vi "DidInit.vi"(8 "ErrorArray":errorcluster[](array[cluster]), 10 "Init?":bool, 11 "Bus":refnum<class "Bus.lvclass">) -> (0 "ErrorArray":errorcluster[](array[cluster]), 3 "Bus":refnum<class "Bus.lvclass">)   [LabVIEW 2014, in "Bus_class.lvlib"]
uses:
  Bus_class.lvlib
  Bus.lvclass
  Typedefs/clDidInit.ctl
  Typedefs/clUserEventType.ctl
  <userlib>/NIST/NISTErrorLib/NISTErrorLib.lvlib
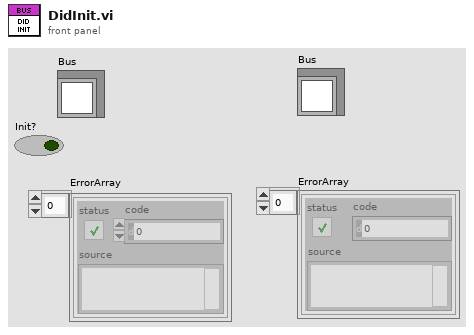
[diagram p1: front panel]
types:
  T1 = typedef "Bus_class.lvlib/clUserEventType.ctl" = cluster{"BusNumber":i8, "Data":variant}
  T2 = typedef "Bus_class.lvlib/clDidInit.ctl" = cluster{"Bus":refnum<vi>, "Init?":bool}
  T3 = typedef "Bus_class.lvlib/clBroadcastEvents.ctl" = cluster{"DidInit":refnum<user-event>, "DidStop":refnum<user-event>}
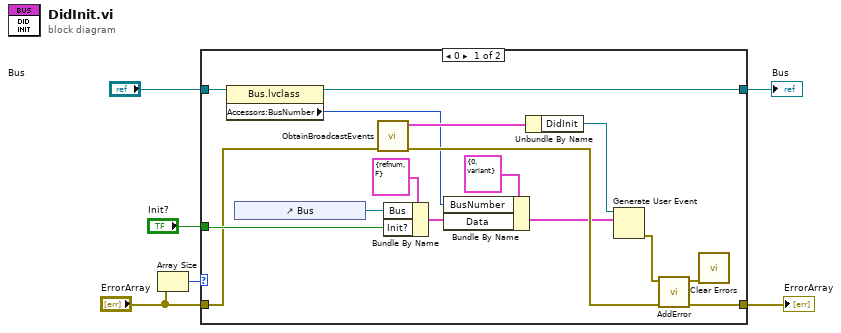
[diagram p0: block diagram]
diagram:
  n1 = Array Size(array="ErrorArray") -> (size(s)=w5:i32)
  n2 = case shown="0" w5 {
    tunnel: "Init?" -> [w19 _]
    tunnel: "ErrorArray" -> [w18 w24]
    tunnel: [w14 w24] -> w3
    tunnel: "Bus" -> [w13 w23]
    tunnel: [w9 w23] -> w1
    frame 0 {
      n3 = property class="Bus.lvclass"(reference=w13) -> (reference out=w9:refnum<class "Bus.lvclass">, "Accessors:BusNumber"=w8:u8)  [unwired: 1 in, 1 out]
      n4 = control-ref of="Bus"() -> (w12:refnum<vi>)
      n5 = call "ObtainBroadcastEvents.vi"("ErrorArray"=w18) -> ("ErrorArray"=w17:errorcluster[], "BusBroadcast"=w22:T3)  [unwired: 9 in]
      n6 = Bundle By Name(cluster=T2 {"Bus"=refnum, "Init?"=FALSE} ("clBusDidInit"), "Bus"=w12, "Init?"=w19) -> (w10:T2)
      n7 = Bundle By Name(cluster=T1 {"BusNumber"=0, "Data"=variant} ("clEventType"), "BusNumber"=w8, "Data"=w10) -> (w7:T1)
      n8 = Unbundle By Name(w22) -> ("DidInit"=w21:refnum<user-event>)
      n9 = Generate User Event(user event=w21, event data cluster=w7) -> (error out=w16:errorcluster)  [unwired: 2 in, 1 out]
      n10 = call <userlib>:"AddError.vi"("ErrorArray"=w17, "error in (no error)"=w16) -> ("ErrorArray"=w14:errorcluster[], "error out"=w15:errorcluster)  [unwired: 8 in]
      n11 = call <vilib>:"Clear Errors.vi"("error in (no error)"=w15) -> ()  [unwired: 5 in, 2 out]
    }
    frame 1, Default {
    }
  }
  "ErrorArray" <- w3
  "Bus" <- w1
